vi "Close Connection.vi"(8 "error in (no error)":errorcluster, 11 "TCPConnection in":refnum<class "TCPConnection.lvclass">) -> (0 "error out":errorcluster, 3 "TCPConnection out":refnum<class "TCPConnection.lvclass">)   [LabVIEW 2013, in "MQTT Server.lvlib" / "TCPConnection.lvclass"]
uses:
  TCPConnection.lvclass
  TCPConnection.lvclass/TCPConnection.ctl
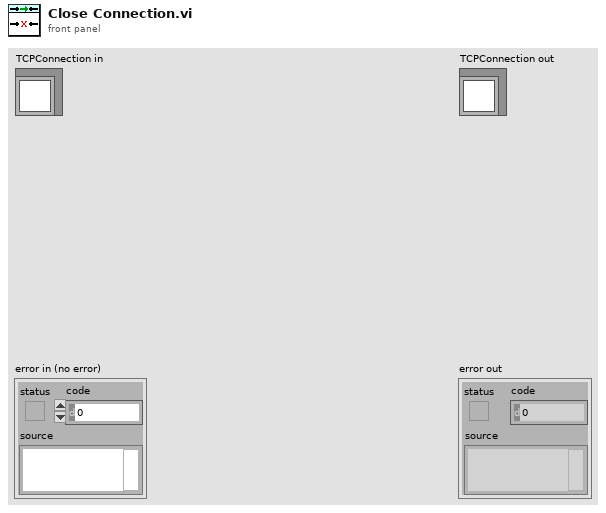
[diagram p1: front panel]
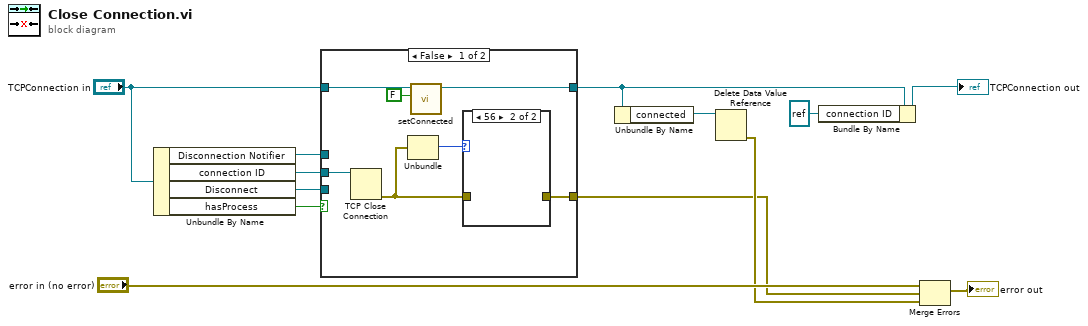
[diagram p0: block diagram]
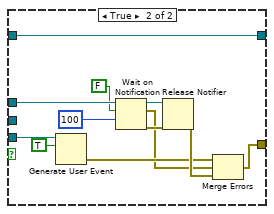
[diagram p3: hidden frame]
diagram:
  n1 = Unbundle By Name("TCPConnection in") -> ("Disconnection Notifier"=w1:refnum<notifier>, "connection ID"=w7:refnum<k5>, "Disconnect"=w5:refnum<user-event>, "hasProcess"=w6:bool)
  n2 = case shown="False" w6 {
    tunnel: w7 -> [w20 _]
    tunnel: w5 -> [_ w32]
    tunnel: [w17 w25] -> w4
    tunnel: "TCPConnection in" -> [w16 w33]
    tunnel: [w15 w33] -> w2
    tunnel: w1 -> [_ w30]
    frame False {
      n3 = TCP Close Connection(connection ID=w20) -> (error out=w18:errorcluster)  [unwired: 2 in, 1 out]
      n4 = Unbundle(w18) -> ("code"=w19:i32)  [unwired: 2 out]
      n5 = call "setConnected.vi"("connected"=FALSE, "TCPConnection in"=w16) -> ("TCPConnection out"=w15:refnum<class "TCPConnection.lvclass">)  [unwired: 8 in, 1 out]
      n6 = case shown="56" w19 {
        tunnel: w18 -> [w21 _]
        tunnel: [w21 _] -> w17
        frame Default {
        }
        frame 56 {
        }
      }
    }
    frame True {
      n7 = Generate User Event(user event=w32, event data cluster=TRUE ("event data")) -> (error out=w23:errorcluster)  [unwired: 2 in, 1 out]
      n8 = Wait on Notification(notifier=w30, ignore previous (F)=FALSE, timeout in ms (-1)=100) -> (notifier out=w26:refnum<notifier>, notification=w22:errorcluster, error out=w27:errorcluster)  [unwired: 1 in, 1 out]
      n9 = Release Notifier(notifier=w26, error in (no error)=w27) -> (error out=w24:errorcluster)  [unwired: 1 in, 2 out]
      n10 = Merge Errors(w23, w22, w24) -> (w25:errorcluster)
    }
  }
  n11 = Unbundle By Name(w2) -> ("connected"=w9:refnum<data-value>)
  n12 = Delete Data Value Reference(data value reference=w9) -> (error out=w8:errorcluster)  [unwired: 1 in, 1 out]
  n13 = Bundle By Name(cluster=w2, "connection ID"=refnum<k5> refnum) -> (→"TCPConnection out":refnum<class "TCPConnection.lvclass">)
  n14 = Merge Errors("error in (no error)", w4, w8) -> (→"error out":errorcluster)
